vi "Read Coils Response.vi"(8 "error in":errorcluster, 10 "modbus data unit in":refnum<class "Modbus Data Unit.lvclass">) -> (0 "error out":errorcluster, 2 "Data":bool[](array[boolean]))   [LabVIEW 2013, in "Modbus Library - Advance.lvlib" / "Master Function Definition.lvclass"]
doc: "Decodes the response for the read coils function."
uses:
  Master Function Definition.lvclass
  Modbus Data Unit/Modbus Data Unit.lvclass
  Modbus Library - Advance.lvlib
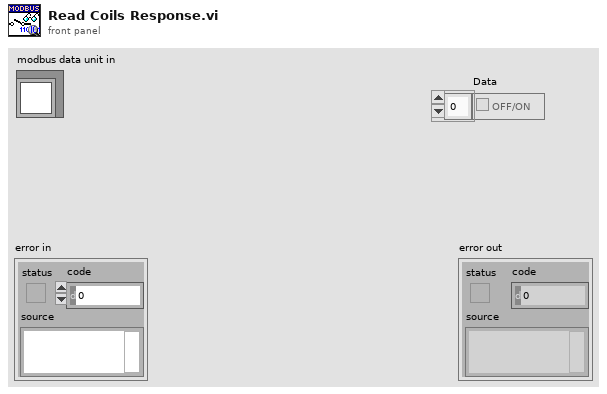
[diagram p1: front panel]
types:
  T1 = typedef "Modbus Library - Advance.lvlib/Modbus Data Unit.lvclass/Function.ctl" = u8
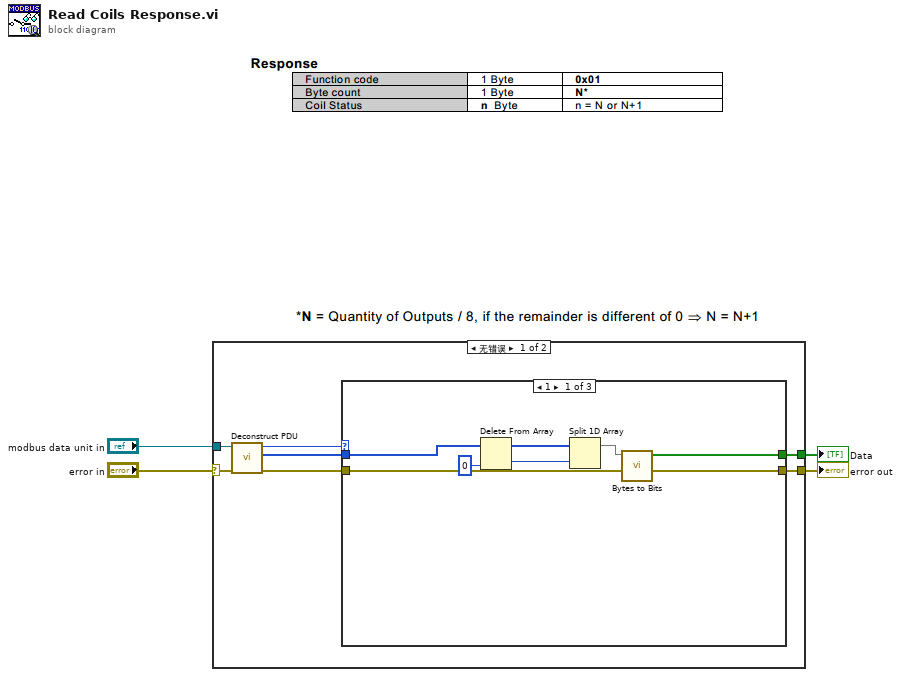
[diagram p0: block diagram]
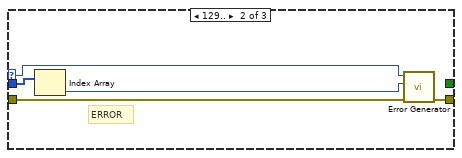
[diagram p2: hidden frame]
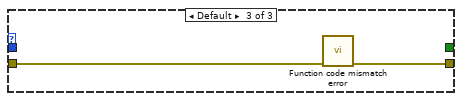
[diagram p3: hidden frame]
diagram:
  n1 = case shown="无错误" "error in" {
    selector: "error in" -> [w5 w26]
    tunnel: [w11 w26] -> w4
    tunnel: "modbus data unit in" -> [w8 _]
    tunnel: [w10 _] -> w2
    frame No Error {
      n2 = call "Deconstruct PDU.vi"("error in"=w5, "modbus data unit in"=w8) -> ("error out"=w7:errorcluster, "data"=w9:u8[], "Function"=w6:T1)  [unwired: 7 in]
      n3 = case shown="1" w6 {
        selector: w6 -> [_ w19 _]
        tunnel: w7 -> [w16 w20 w25]
        tunnel: w9 -> [w18 w23 _]
        tunnel: [w16 w22 w24] -> w11
        tunnel: [w17 _ _] -> w10
        frame 1 {
          n4 = Delete From Array(array=w18, index=0) -> (deleted portion=w14:u8, array with subset deleted=w13:u8[])  [unwired: 1 in]
          n5 = Split 1D Array(array=w13, index=w14) -> (first subarray=w15:u8[])  [unwired: 1 out]
          n6 = call "Bytes to Bits.vi"("Bytes"=w15) -> ("Bits"=w17:bool[])  [unwired: 10 in]
        }
        frame 129.. {
          # "ERROR"
          n7 = Index Array(array=w23) -> (element=w21:u8)  [unwired: 1 in]
          n8 = call "Error Generator.vi"("error in"=w20, "data return (error code)"=w21, "function return"=w19) -> ("error out"=w22:errorcluster)  [unwired: 8 in]
        }
        frame Default {
          n9 = call "Function code mismatch error.vi"("error in (no error)"=w25) -> ("error out"=w24:errorcluster)  [unwired: 10 in]
        }
      }
    }
    frame Error {
    }
  }
  "error out" <- w4
  "Data" <- w2
